vi "Newton Raphson Zero Finder (VI).vi"(6 "data":variant, 7 "accuracy":dbl=1e-08 format="%.2e", 8 "f(x)":T1, 9 "end":dbl=1.0 format="%.2f", 10 "start":dbl format="%.2f", 11 "h":dbl=1e-08 format="%.2e") -> (0 "error":i32, 1 "ticks":u32, 2 "f(zero)":dbl format="%.2f", 3 "zero":dbl format="%.2f")   [LabVIEW 2024, in "NI_Gmath.lvlib"]
doc: "<p>Determines a zero of a 1D function close to two points with the help of the derivative of this 1D function. The two values form a search limit for the unknown zero of the 1D function. You must <a href=\"nihelplauncher://docs/csh?context=lvcore_lvhowto_selectingdefaultinstpolyvi\">manually select the polymorphic instance</a> to use.</p>"
uses:
  NI_Gmath.lvlib
  functionRefnum.ctl
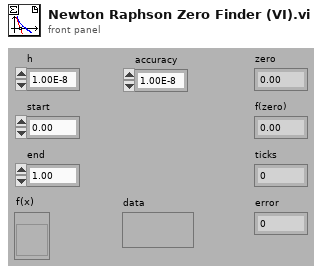
[diagram p1: front panel]
types:
  T1 = typedef "NI_Gmath.lvlib/functionRefnum.ctl" = refnum<vi>
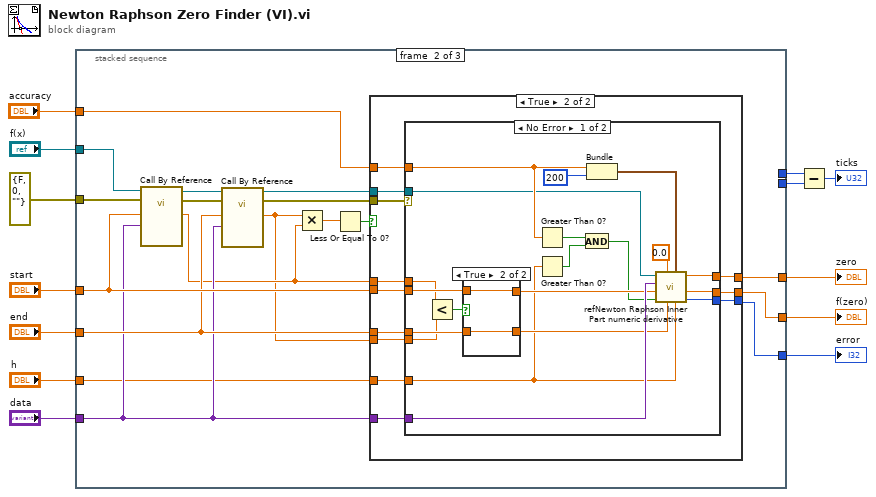
[diagram p0: block diagram]
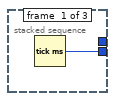
[diagram p2: hidden frame]
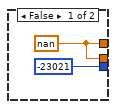
[diagram p3: hidden frame]
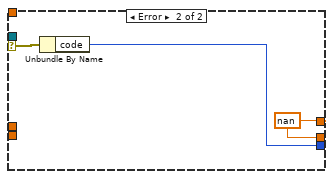
[diagram p5: hidden frame]
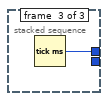
[diagram p6: hidden frame]
diagram:
  n1 = stacked-sequence {
    tunnel: [_ w31 _] -> w13
    tunnel: [_ w30 _] -> w12
    tunnel: [_ w29 _] -> w11
    tunnel: "f(x)" -> [_ w22 _]
    tunnel: "data" -> [_ w24 _]
    tunnel: "start" -> [_ w27 _]
    tunnel: "end" -> [_ w25 _]
    tunnel: [w14 _ _] -> w6
    tunnel: [_ _ w74] -> w5
    tunnel: errorcluster {"status"=FALSE, "code"=0, "source"=""} ("error in (no error)") -> [_ w28 _]
    tunnel: "accuracy" -> [_ w16 _]
    tunnel: "h" -> [_ w15 _]
    frame #0 {
      n2 = Tick Count (ms)() -> (millisecond timer value=w14:u32)
    }
    frame #1 {
      n3 = call-by-ref "?"(reference=w22, error in=w28, "Variant"=w24, "x"=w27) -> (reference out=w26:T1, error out=w18:errorcluster, 2:"f(x)"=w23:dbl)  [unwired: 3 in]
      n4 = call-by-ref "?"(reference=w26, error in=w18, "Variant"=w24, "x"=w25) -> (reference out=w21:T1, error out=w17:errorcluster, 2:"f(x)"=w19:dbl)  [unwired: 3 in]
      n5 = Multiply(x=w19, y=w23) -> (x*y=w32:dbl)
      n6 = Less Or Equal To 0?(x=w32) -> (x <= 0?=w20:bool)
      n7 = case shown="True" w20 {
        tunnel: w27 -> [_ w46]
        tunnel: w25 -> [_ w45]
        tunnel: [w34 w42] -> w31
        tunnel: [w34 w41] -> w30
        tunnel: [-23021 w40] -> w29
        tunnel: w23 -> [_ w44]
        tunnel: w19 -> [_ w43]
        tunnel: w21 -> [_ w39]
        tunnel: w24 -> [_ w38]
        tunnel: w17 -> [_ w37]
        tunnel: w16 -> [_ w36]
        tunnel: w15 -> [_ w35]
        frame False {
          w34 = nan
        }
        frame True {
          n8 = case shown="No Error" w37 {
            selector: w37 -> [_ w73]
            tunnel: w46 -> [w63 _]
            tunnel: w45 -> [w62 _]
            tunnel: w44 -> [w61 _]
            tunnel: w43 -> [w47 _]
            tunnel: [w56 w71] -> w42
            tunnel: [w55 w71] -> w41
            tunnel: [w54 w72] -> w40
            tunnel: w39 -> [w48 _]
            tunnel: w38 -> [w59 _]
            tunnel: w36 -> [w50 _]
            tunnel: w35 -> [w49 _]
            frame No Error {
              n9 = Less?(x=w61, y=w47) -> (x < y?=w64:bool)
              n10 = case shown="True" w64 {
                tunnel: w63 -> [w68 w70]
                tunnel: w62 -> [w67 w69]
                tunnel: [w67 w70] -> w58
                tunnel: [w68 w69] -> w53
                frame False {
                }
                frame True {
                }
              }
              n11 = Greater Than 0?(x=w50) -> (x > 0?=w66:bool)
              n12 = Greater Than 0?(x=w49) -> (x > 0?=w65:bool)
              n13 = And(x=w66, y=w65) -> (x .and. y?=w57:bool)
              n14 = Bundle("accuracy"=w50, 200) -> (w51:cluster{"accuracy":dbl, i32})  [unwired: 1 out]
              n15 = call "refNewton Raphson Inner Part numeric derivative.vi"("h"=w49, "NR Settings"=w51, "end/start"=w53, "level"=0.0, "case"=w57, "start/end"=w58, "Variant"=w59, "function refnum"=w48) -> ("error"=w54:i32, "f(zero)"=w55:dbl, "zero"=w56:dbl)  [unwired: 1 out]
            }
            frame Error {
              w71 = nan ("zero")
              n16 = Unbundle By Name(w73) -> ("code"=w72:i32)
            }
          }
        }
      }
    }
    frame #2 {
      n17 = Tick Count (ms)() -> (millisecond timer value=w74:u32)
    }
  }
  "zero" <- w13
  "f(zero)" <- w12
  "error" <- w11
  n18 = Subtract(x=w5, y=w6) -> (x-y=→"ticks":u32)
